vi "New Execution.vi"(0 "Execution Options (Default)":T1, 11 "error in (no error)":errorcluster) -> (4 "Session Handle out":T2, 15 "error out":errorcluster)   [LabVIEW 2020, in "TSS.lvlib" / "Execution.lvclass"]
uses:
  Execution.lvclass
  Typedefs/Session Handle.ctl
  Execution Options.ctl
  Engine/Engine.lvclass
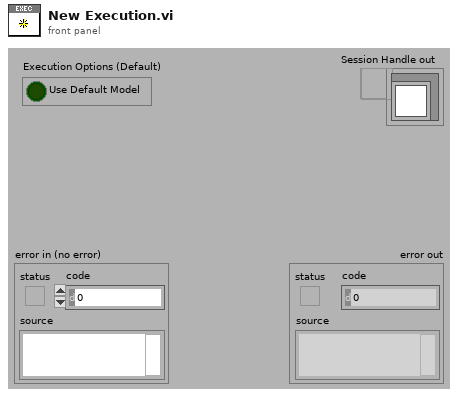
[diagram p1: front panel]
types:
  T1 = typedef "TSS.lvlib/Execution.lvclass/Execution Options.ctl" = cluster{"Use Default Model":bool}
  T2 = typedef "TSS.lvlib/Execution.lvclass/Session Handle.ctl" = refnum<data-value>
  T3 = typedef "TSS.lvlib/Engine.lvclass/Session Handle.ctl" = refnum<data-value>
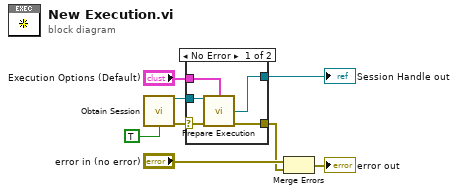
[diagram p0: block diagram]
diagram:
  n1 = call "Obtain Session.vi"("Error to Create? (F)"=TRUE) -> ("Session Handle"=w5:T3, "error out"=w6:errorcluster)  [unwired: 12 in, 1 out]
  n2 = case shown="No Error" w6 {
    selector: w6 -> [w12 w14]
    tunnel: w5 -> [w13 _]
    tunnel: "Execution Options (Default)" -> [w11 _]
    tunnel: [w10 _] -> w3
    tunnel: [w9 w14] -> w1
    frame No Error {
      n3 = call "Prepare Execution.vi"("Session Handle in"=w13, "Options (Default)"=w11, "error in (no error)"=w12) -> ("Execution"=w10:T2, "error out"=w9:errorcluster)  [unwired: 10 in, 1 out]
    }
    frame Error {
    }
  }
  "Session Handle out" <- w3
  n4 = Merge Errors("error in (no error)", w1) -> (→"error out":errorcluster)
